vi "Initialize.vi"(5 "Plugins":refnum<class "Plugin.lvclass">[](array[class]), 6 "Enable":bool, 7 "Project":refnum<class "Project.lvclass">, 8 "error in (no error)":errorcluster, 9 "Container":refnum<vi>, 10 "Index":u8, 11 "Execution in":refnum<data-value>) -> (0 "error out":errorcluster, 3 "Execution out":refnum<data-value>)   [LabVIEW 2015, in "Execution.lvclass"]
uses:
  Execution.lvclass
  Project.lvclass
  Plugin.lvclass
  EXECUTION_UI_QUEUE_DATA.ctl
  EXECUTION_UI_MSG.ctl
  BACKGROUND_CONTROL_MSG_TYPEDEF.ctl
  EXECUTION_STATUS.ctl
  EXECUTION_CTRL_QUEUE_DATA.ctl
  EXECUTION_CTRL_MSG.ctl
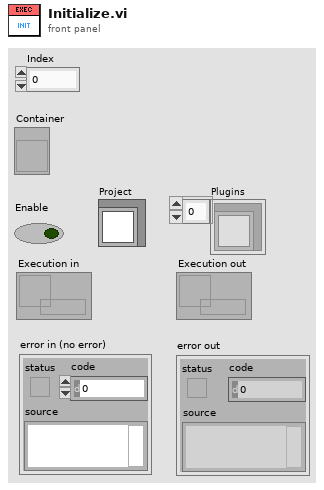
[diagram p1: front panel]
types:
  T1 = typedef "Execution.lvclass/EXECUTION_CTRL_QUEUE_DATA.ctl" = cluster{"Msg":T2, "Data":variant}
  T2 = typedef "Execution.lvclass/EXECUTION_CTRL_MSG.ctl" = enum16{"EXECUTION_START", "EXECUTION_END", "EXECUTION_LOOP", "APPLICATION_STOP"}
  T3 = typedef "Execution.lvclass/EXECUTION_STATUS.ctl" = enum16{"Initializing ", "Disable", "Ready", "Running", "Finished"}
  T4 = typedef "Execution.lvclass/BACKGROUND_CONTROL_MSG_TYPEDEF.ctl" = cluster{"Target":string, "Msg":string, "Data":variant}
  T5 = typedef "Execution.lvclass/EXECUTION_UI_QUEUE_DATA.ctl" = cluster{"Msg":T6, "Data":variant}
  T6 = typedef "Execution.lvclass/EXECUTION_UI_MSG.ctl" = enum16{"EXECUTION_STATUS", "INIT_UI", "DUT_UPDATE", "BOTTOM_PANEL_UPDATE", "TOP_PANEL_UPDATE", "STEP_START", "STEP_END", "DISPLAY_RESULT", "APPLICATION_END"}
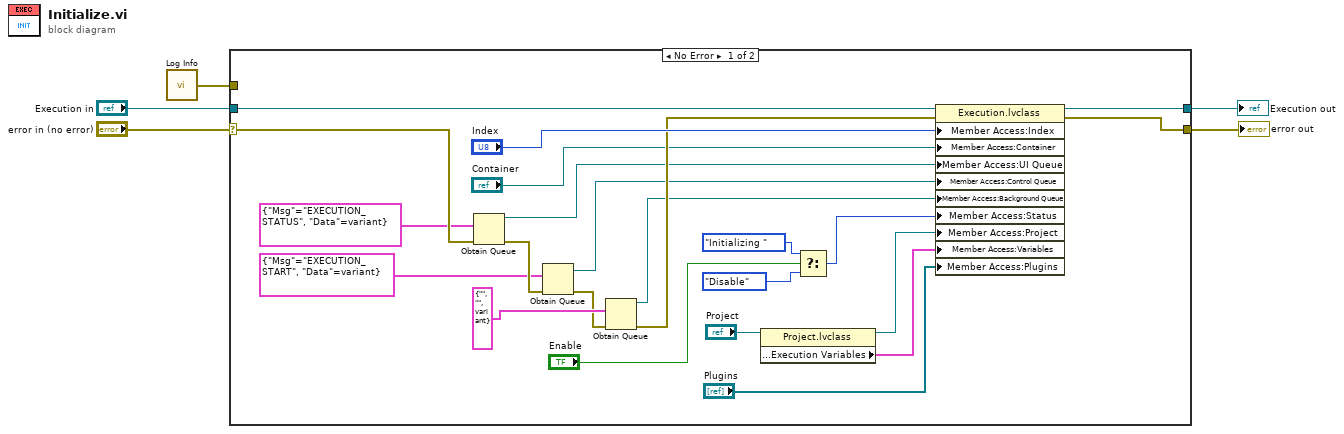
[diagram p0: block diagram]
diagram:
  n1 = call "Log Info.vi"() -> ("error out"=w1:errorcluster)  [unwired: 5 in]
  n2 = case shown="No Error" "error in (no error)" {
    selector: "error in (no error)" -> [w27 w30]
    tunnel: [w18 w30] -> w4
    tunnel: [w26 w29] -> w2
    tunnel: "Execution in" -> [w28 w29]
    tunnel: w1 -> [_ _]
    frame No Error {
      n3 = Obtain Queue(element data type=T5 {"Msg"=enum."EXECUTION_STATUS", "Data"=variant} ("UI_MSG"), error in (no error)=w27) -> (queue out=w12:refnum<queue>, error out=w15:errorcluster)  [unwired: 3 in, 1 out]
      n4 = Obtain Queue(element data type=T1 {"Msg"=enum."EXECUTION_START", "Data"=variant} ("Ctrl Msg"), error in (no error)=w15) -> (queue out=w10:refnum<queue>, error out=w14:errorcluster)  [unwired: 3 in, 1 out]
      n5 = Obtain Queue(element data type=T4 {"Target"="", "Msg"="", "Data"=variant} ("Cluster"), error in (no error)=w14) -> (queue out=w16:refnum<queue>, error out=w24:errorcluster)  [unwired: 3 in, 1 out]
      n6 = property class="Project.lvclass"(reference="Project") -> (reference out=w8:refnum<class "Project.lvclass">, "Member Access:Execution Variables"=w7:cluster{"Name":string, "Value":variant}[])  [unwired: 1 in, 1 out]
      n7 = Select(t=EXECUTION_STATUS."Initializing " ("Status"), s="Enable", f=EXECUTION_STATUS."Disable" ("Status")) -> (s? t:f=w17:T3)
      n8 = property class="Execution.lvclass"(reference=w28, error in=w24, "Member Access:Index"="Index", "Member Access:Container"="Container", "Member Access:UI Queue"=w12, "Member Access:Control Queue"=w10, "Member Access:Background Queue"=w16, "Member Access:Status"=w17, "Member Access:Project"=w8, "Member Access:Variables"=w7, "Member Access:Plugins"="Plugins") -> (reference out=w26:refnum<data-value>, error out=w18:errorcluster)
    }
    frame Error {
    }
  }
  "error out" <- w4
  "Execution out" <- w2
